vi "Read Lockin Class.vi"(8 "error in (no error)":errorcluster, 11 "UI.Lockin in":refnum<class "UI.Lockin.lvclass">) -> (0 "error out":errorcluster, 2 "system":refnum<class "multichannel-lockin.lvclass">, 3 "UI.Lockin out":refnum<class "UI.Lockin.lvclass">)   [LabVIEW 2019, in "UI.Lockin.lvclass"]
uses:
  UI.Lockin.lvclass
  lockin/multichannel-lockin.lvclass
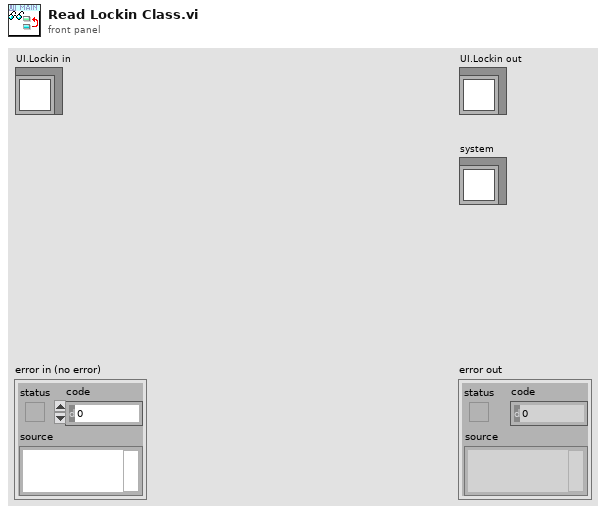
[diagram p1: front panel]
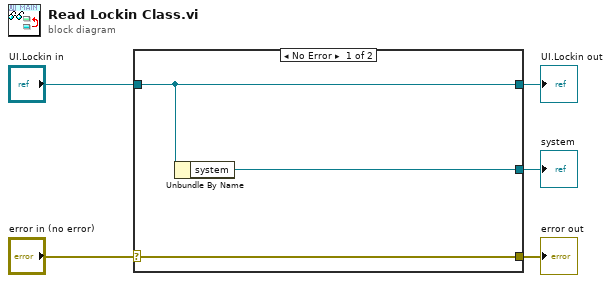
[diagram p0: block diagram]
diagram:
  n1 = case shown="No Error" "error in (no error)" {
    selector: "error in (no error)" -> [w8 w9]
    tunnel: [w8 w9] -> w4
    tunnel: [w7 w10] -> w2
    tunnel: "UI.Lockin in" -> [w7 w10]
    tunnel: [w6 _] -> w1
    frame No Error {
      n2 = Unbundle By Name(w7) -> ("system"=w6:refnum<class "multichannel-lockin.lvclass">)
    }
    frame Error {
    }
  }
  "error out" <- w4
  "UI.Lockin out" <- w2
  "system" <- w1
